vi "svx_Polar_Autoscale.vi"(8 "State":T2={"Property Name"=[], "Container bounds"={"Width"=550, "Height"=250}, "Scale range"={"Maximum"=1.0, "Increment"=1.0}, "PointIdx"=0, "Marker list"=[], "Color settings"={"Arrow color"=16860, "Magnitude major grid"=13816530, "Magnitude minor grid"=16777216, "Phase grid"=13816530, "Phase scale marker text"=0}, "Magnitude scale name"="Magnitude", "Magnitude scale format string"="%#.2e", "MagnitudeScale:Visible"=TRUE, "MagnitudeScaleLabel:Visible"=TRUE, "PhaseScale:Visible"=TRUE, "Marker:Visible"=TRUE, "Cursor:Visible"=FALSE, "CursorName:Visible"=TRUE, "Autoscale"=TRUE, "Marker color"=16860, "Line color"=16711680, "Cursor color"=16711680, "Magnitude scale marker color"=0, "Plot.Line Style"=0, "Plot.Line Width"=0, "Plot.Point Style"=0, "Cursor.Line Style"=0, "Cursor.Line Width"=0, "Cursor.Point Style"=0, "Cursor.Style"=4, "Marker.Point Style"=2, "Point/fill color"=16711680, "Background color"=16777225, "Cursor name"="", "Cursor Release"=refnum, "Scale Range Change"=refnum, "data size(s)"=[], "Selectors:Visible"=TRUE, "Selector:ring Strings"={"Selector:Custom Strings"=FALSE, "Selector:Row Strings []"=[], "Selector:Column Strings []"=[], "User:Row Strings []"=[], "User:Column Strings []"=[]}, "Lock Cursor Info Position"=FALSE, "CursLoc"={"magnitude"=0.0, "phase"=0.0, "time/rev/RPM"=0.0}, "Plot Area:Position"={"Left"=0, "Top"=0}, "Plot Area:Size"={"Width"=0, "Height"=0}, "Marker.Style"=0, "Indication Arcs"=[], "Arc.Selector"=0, "customized marker"=[], "tree Width"=0, " Parents Tags"=[], "Children Tags"=[], "open?"=[], "index"=[{"row index"=0, "column index"=0}], "Label"="", "custom strings changed"=FALSE, "Owning VI"=refnum, "Legend BG color"=16777225, "Legend font color"=0, "column Width"=203, "attribute"=variant}, 9 "polar plot":T1, 10 "z scale graph":refnum<vi>, 11 "Polar Plot":refnum<vi>) -> (0 "State out":T2={"Property Name"=[], "Container bounds"={"Width"=550, "Height"=250}, "Scale range"={"Maximum"=1.0, "Increment"=1.0}, "PointIdx"=0, "Marker list"=[], "Color settings"={"Arrow color"=16860, "Magnitude major grid"=13816530, "Magnitude minor grid"=16777216, "Phase grid"=13816530, "Phase scale marker text"=0}, "Magnitude scale name"="Magnitude", "Magnitude scale format string"="%#.2e", "MagnitudeScale:Visible"=TRUE, "MagnitudeScaleLabel:Visible"=TRUE, "PhaseScale:Visible"=TRUE, "Marker:Visible"=TRUE, "Cursor:Visible"=FALSE, "CursorName:Visible"=TRUE, "Autoscale"=TRUE, "Marker color"=16860, "Line color"=16711680, "Cursor color"=16711680, "Magnitude scale marker color"=0, "Plot.Line Style"=0, "Plot.Line Width"=0, "Plot.Point Style"=0, "Cursor.Line Style"=0, "Cursor.Line Width"=0, "Cursor.Point Style"=0, "Cursor.Style"=4, "Marker.Point Style"=2, "Point/fill color"=16711680, "Background color"=16777225, "Cursor name"="", "Cursor Release"=refnum, "Scale Range Change"=refnum, "data size(s)"=[], "Selectors:Visible"=TRUE, "Selector:ring Strings"={"Selector:Custom Strings"=FALSE, "Selector:Row Strings []"=[], "Selector:Column Strings []"=[], "User:Row Strings []"=[], "User:Column Strings []"=[]}, "Lock Cursor Info Position"=FALSE, "CursLoc"={"magnitude"=0.0, "phase"=0.0, "time/rev/RPM"=0.0}, "Plot Area:Position"={"Left"=0, "Top"=0}, "Plot Area:Size"={"Width"=0, "Height"=0}, "Marker.Style"=0, "Indication Arcs"=[], "Arc.Selector"=0, "customized marker"=[], "tree Width"=0, " Parents Tags"=[], "Children Tags"=[], "open?"=[], "index"=[{"row index"=0, "column index"=0}], "Label"="", "custom strings changed"=FALSE, "Owning VI"=refnum, "Legend BG color"=16777225, "Legend font color"=0, "column Width"=203, "attribute"=variant} caption="State", 1 "redraw scale?":bool, 2 "z scale graph ref out":refnum<vi>, 3 "Polar Plot ref out":refnum<vi>)   [LabVIEW 2017, in "SVX Polar Plot.xctl"]
uses:
  <vilib>/addons/_XControls/Polar Plot/SVX Polar Plot.xctl
  <vilib>/addons/_XControls/Polar Plot/subVIs/svx_Polar_Plot_Internal_State.ctl
  <vilib>/addons/_XControls/Polar Plot/subVIs/svx_Polar_Indication_Arcs.ctl
  <vilib>/addons/_XControls/Polar Plot/subVIs/svx_Polar_Customized_Markers.ctl
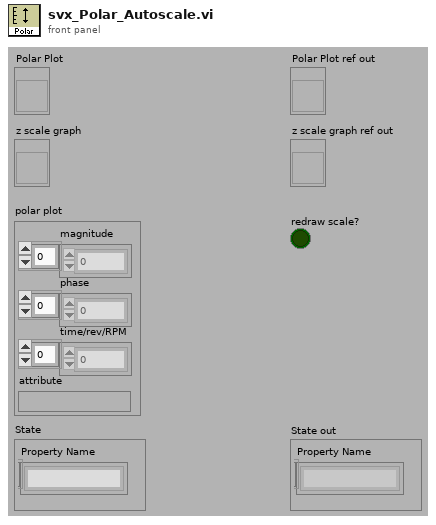
[diagram p1: front panel]
types:
  T1 = cluster{"magnitude":dbl[], "phase":dbl[], "time/rev/RPM":dbl[], "attribute":variant}
  T2 = typedef "SVX Polar Plot.xctl/svx_Polar_Plot_Internal_State.ctl" = cluster{"Property Name":string[], "Container bounds":cluster{"Width":u32, "Height":u32}, "Scale range":cluster{"Maximum":dbl, "Increment":dbl}, "PointIdx":i32, "Marker list":cluster{"Name":string, "Color":u32, "Style":u8, "Point Style":u8, "Name Visible":bool, "Allow Drag":bool, "Annotation Mode":u32, "Plot":i32, "Index":i32, "Position":cluster{"X":dbl, "Y":dbl}, "X Scale":u32, "Y Scale":u32, "Show Arrow":bool, "Lock Name":bool, "Plot Area":i32, "Label Offset":cluster{"X":dbl, "Y":dbl}}[], "Color settings":cluster{"Arrow color":u32, "Magnitude major grid":u32, "Magnitude minor grid":u32, "Phase grid":u32, "Phase scale marker text":u32}, "Magnitude scale name":string, "Magnitude scale format string":string, "MagnitudeScale:Visible":bool, "MagnitudeScaleLabel:Visible":bool, "PhaseScale:Visible":bool, "Marker:Visible":bool, "Cursor:Visible":bool, "CursorName:Visible":bool, "Autoscale":bool, "Marker color":u32, "Line color":u32, "Cursor color":u32, "Magnitude scale marker color":u32, "Plot.Line Style":i32, "Plot.Line Width":i32, "Plot.Point Style":i32, "Cursor.Line Style":i32, "Cursor.Line Width":i32, "Cursor.Point Style":i32, "Cursor.Style":i32, "Marker.Point Style":i32, "Point/fill color":u32, "Background color":u32, "Cursor name":string, "Cursor Release":refnum<user-event>, "Scale Range Change":refnum<user-event>, "data size(s)":i32[], "Selectors:Visible":bool, "Selector:ring Strings":cluster{"Selector:Custom Strings":bool, "Selector:Row Strings []":string[], "Selector:Column Strings []":string[], "User:Row Strings []":string[], "User:Column Strings []":string[]}, "Lock Cursor Info Position":bool, "CursLoc":cluster{"magnitude":dbl, "phase":dbl, "time/rev/RPM":dbl}, "Plot Area:Position":cluster{"Left":i32, "Top":i32}, "Plot Area:Size":cluster{"Width":u32, "Height":u32}, "Marker.Style":i32, "Indication Arcs":T3, "Arc.Selector":u16, "customized marker":T4, "tree Width":u32, " Parents Tags":string[], "Children Tags":string[], "open?":bool[], "index":cluster{"row index":i32, "column index":i32}[], "Label":string, "custom strings changed":bool, "Owning VI":refnum<vi>, "Legend BG color":u32, "Legend font color":u32, "column Width":u32, "attribute":variant}
  T3 = typedef "SVX Polar Plot.xctl/svx_Polar_Indication_Arcs.ctl" = cluster{"Name":string, "Start radius":dbl, "End radius":dbl, "Line Style":i32, "Line Width":i32, "Border color":u32, "Fill color":u32, "Start angle":i16, "End angle":i16, "Visible":bool}[]
  T4 = typedef "SVX Polar Plot.xctl/svx_Polar_Customized_Markers.ctl" = cluster{"Name":string, "Color":u32, "Style":u8, "Point Style":u8, "Name Visible":bool, "Allow Drag":bool, "Annotation Mode":u32, "Plot":i32, "Index":i32, "Position":cluster{"Magnitude":dbl, "Phase":dbl}, "X Scale":u32, "Y Scale":u32, "Show Arrow":bool, "Lock Name":bool, "Plot Area":i32, "Label Offset":cluster{"Magnitude":dbl, "Phase":dbl}}[]
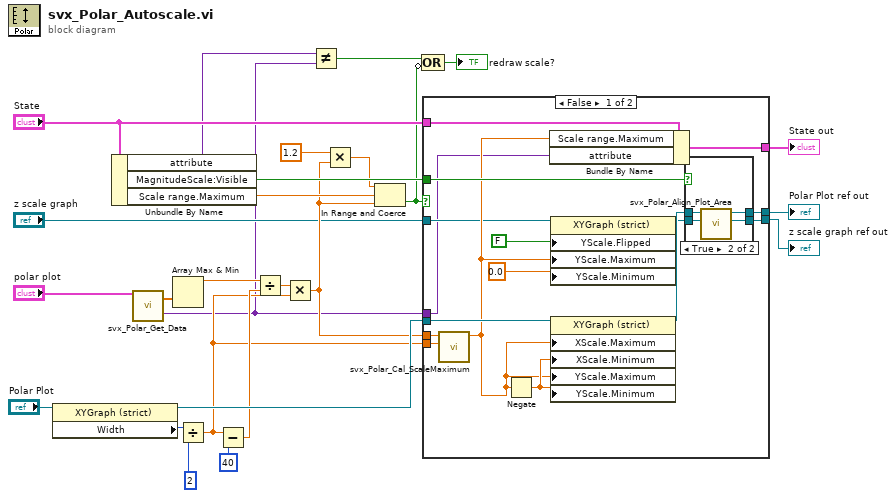
[diagram p0: block diagram]
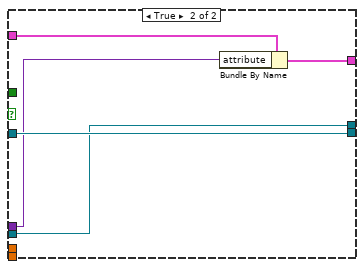
[diagram p3: hidden frame]
diagram:
  n1 = property class="XYGraph (strict)"(reference="Polar Plot") -> (reference out=w21:refnum<vi>, "Width"=w13:u32)  [unwired: 1 in, 1 out]
  n2 = Unbundle By Name("State") -> ("attribute"=w7:variant, "MagnitudeScale:Visible"=w23:bool, "Scale range.Maximum"=w25:dbl)
  n3 = call <vilib>:"svx_Polar_Get_Data.vi"("polar plot"="polar plot") -> ("magnitude"=w22:dbl[], "attribute"=w6:variant)  [unwired: 13 in, 4 out]
  n4 = Array Max & Min(array=w22) -> (max value=w20:dbl)  [unwired: 3 out]
  n5 = Divide(x=w13, y=u32 2) -> (x/y=w12:dbl)
  n6 = Subtract(x=w12, y=u32 40) -> (x-y=w19:dbl)
  n7 = Divide(x=w20, y=w19) -> (x/y=w18:dbl)
  n8 = Multiply(x=w18, y=w12) -> (x*y=w10:dbl)
  n9 = Not Equal?(x=w7, y=w6) -> (x != y?=w4:bool)
  n10 = Multiply(x=1.2 ("y"), y=w10) -> (x*y=w15:dbl)
  n11 = In Range and Coerce(upper limit=w15, x=w25, lower limit=w10) -> (In Range?=w5:bool)  [unwired: 1 out]
  n12 = Compound Arithmetic op=OR(w4, invert w5) -> (→"redraw scale?":bool)
  n13 = case shown="False" w5 {
    tunnel: "State" -> [w42 w51]
    tunnel: [w41 w49] -> w24
    tunnel: w23 -> [w39 _]
    tunnel: w21 -> [w38 w52]
    tunnel: w12 -> [w31 _]
    tunnel: w10 -> [w32 _]
    tunnel: [w30 w52] -> w1
    tunnel: [w29 w53] -> w9
    tunnel: "z scale graph" -> [w28 w53]
    tunnel: w6 -> [w27 w50]
    frame False {
      n14 = call <vilib>:"svx_Polar_Cal_ScaleMaximum.vi"("scale width"=w31, "original maximum"=w32) -> ("best maximum"=w33:dbl)  [unwired: 9 in]
      n15 = Negate(x=w33) -> (-x=w37:dbl)
      n16 = Bundle By Name(cluster=w42, "Scale range.Maximum"=w33, "attribute"=w27) -> (w41:T2)
      n17 = property class="XYGraph (strict)"(reference=w28, "YScale.Flipped"=FALSE ("Y Scale.Flipped"), "YScale.Maximum"=w33, "YScale.Minimum"=0.0 ("Minimum")) -> (reference out=w35:refnum<vi>)  [unwired: 1 in, 1 out]
      n18 = property class="XYGraph (strict)"(reference=w38, "XScale.Maximum"=w33, "XScale.Minimum"=w37, "YScale.Maximum"=w33, "YScale.Minimum"=w37) -> (reference out=w40:refnum<vi>)  [unwired: 1 in, 1 out]
      n19 = case shown="True" w39 {
        tunnel: w40 -> [w44 w48]
        tunnel: w35 -> [w43 w47]
        tunnel: [w44 w46] -> w30
        tunnel: [w43 w45] -> w29
        frame False {
        }
        frame True {
          n20 = call <vilib>:"svx_Polar_Align_Plot_Area.vi"("z scale graph ref in"=w47, "Polar Plot ref in"=w48) -> ("z scale graph ref out"=w45:refnum<vi>, "Polar Plot ref out"=w46:refnum<vi>)  [unwired: 8 in]
        }
      }
    }
    frame True {
      n21 = Bundle By Name(cluster=w51, "attribute"=w50) -> (w49:T2)
    }
  }
  "State out" <- w24
  "z scale graph ref out" <- w9
  "Polar Plot ref out" <- w1
